vi "Configure Control (Digital).vi"(8 "error in":errorcluster, 10 "control":refnum<vi>, 11 "NT Scalar (Numeric) in":refnum<class "NT Scalar (Numeric).lvclass">) -> (0 "error out":errorcluster, 2 "control out":refnum<vi>, 3 "NT Scalar (Numeric) out":refnum<class "NT Scalar (Numeric).lvclass">)   [LabVIEW 2020, in "PV Access.lvlib" / "PV Data.lvlib" / "NT Scalar (Numeric).lvclass"]
doc: "Set the description, control limits, format and precision of <B>control</B> from the value's metadata."
uses:
  NT Scalar (Numeric).lvclass
  NT Scalar (Numeric).lvclass/NT Scalar (Numeric).ctl
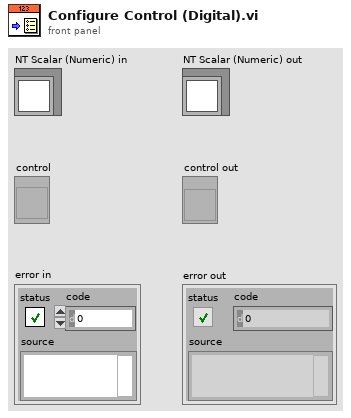
[diagram p1: front panel]
types:
  T1 = typedef "PV Access.lvlib/PV Data.lvlib/Display Form.ctl" = enum32{"Default", "String", "Binary", "Decimal", "Hex", "Exponential", "Engineering"}
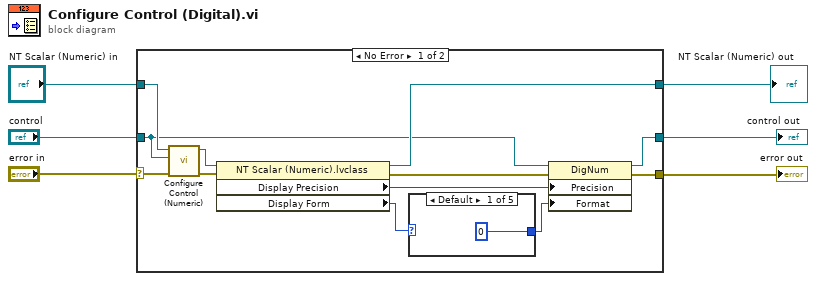
[diagram p0: block diagram]
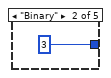
[diagram p2: hidden frame]
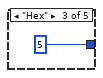
[diagram p3: hidden frame]
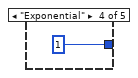
[diagram p4: hidden frame]
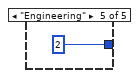
[diagram p5: hidden frame]
diagram:
  n1 = case shown="No Error" "error in" {
    selector: "error in" -> [w13 w25]
    tunnel: [w14 w26] -> w6
    tunnel: "NT Scalar (Numeric) in" -> [w12 w26]
    tunnel: [w10 w25] -> w3
    tunnel: [w8 w24] -> w2
    tunnel: "control" -> [w7 w24]
    frame No Error {
      n2 = call "Configure Control (Numeric).vi"("error in"=w13, "control"=w7, "NT Scalar (Numeric) in"=w12) -> ("error out"=w9:errorcluster, "NT Scalar (Numeric) out"=w11:refnum<class "NT Scalar (Numeric).lvclass">)  [unwired: 6 in, 1 out]
      n3 = property class="NT Scalar (Numeric).lvclass"(reference=w11, error in=w9) -> (reference out=w14:refnum<class "NT Scalar (Numeric).lvclass">, error out=w17:errorcluster, "Display Precision"=w16:i32, "Display Form"=w15:T1)
      n4 = case shown="Default" w15 {
        tunnel: [u8 0 u8 3 u8 5 u8 1 u8 2] -> w18
        frame Default {
        }
        frame "Binary" {
        }
        frame "Hex" {
        }
        frame "Exponential" {
        }
        frame "Engineering" {
        }
      }
      n5 = property on="Property Node" class="DigNum"(reference=w7, error in=w17, "Precision"=w16, "Format"=w18) -> (reference out=w8:refnum<vi>, error out=w10:errorcluster)
    }
    frame Error {
    }
  }
  "error out" <- w3
  "NT Scalar (Numeric) out" <- w6
  "control out" <- w2
